vi "Trapezoid Logic.vi"(8 "Total Power":dbl, 9 "Ramp Distance":dbl, 10 "Stop Distance":dbl, 11 "Current \nDistance":dbl(slide) scale=0.0..20.0) -> (2 "Speed":dbl)   [LabVIEW 2013]
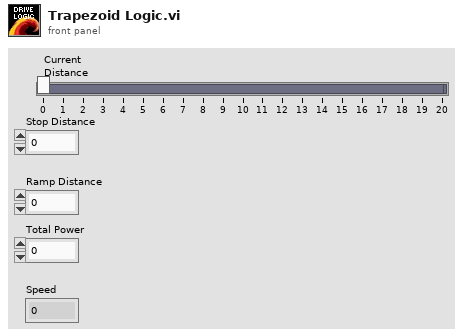
[diagram p1: front panel]
types:
  T1 = enum16{"End Ramp", "Continue Ramp", "Start Ramp"}
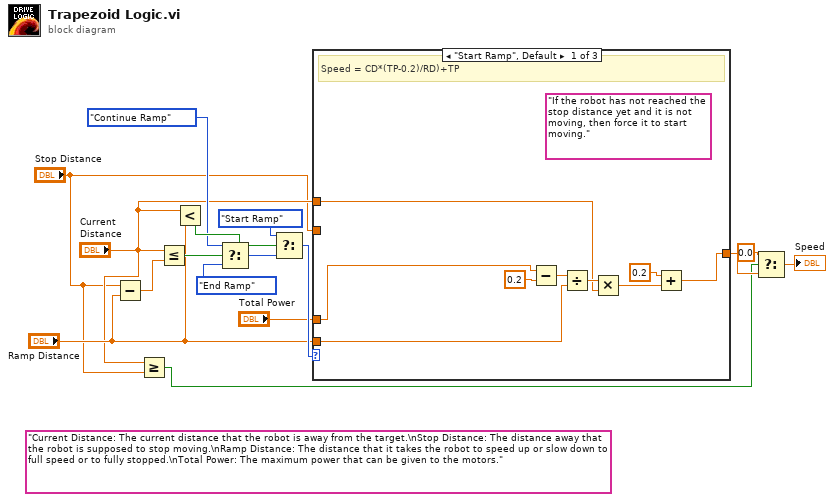
[diagram p0: block diagram]
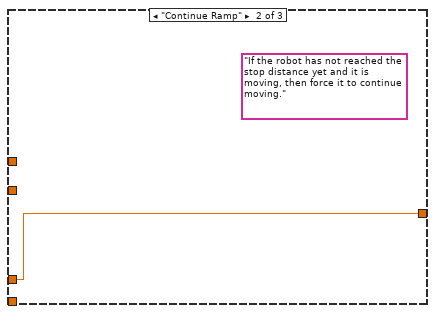
[diagram p2: hidden frame]
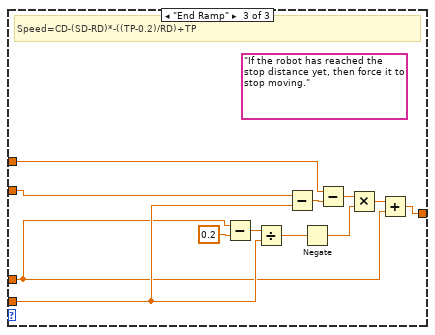
[diagram p3: hidden frame]
diagram:
  (unwired) "Current Distance: The current distance that the robot is away from the target.\nStop Distance: The distance away that the robot is supposed to stop moving.\nRamp Distance: The distance that it takes the robot to speed up or slow down to full speed or to fully stopped.\nTotal Power: The maximum power that can be given to the motors."
  n1 = Subtract(x="Stop Distance", y="Ramp Distance") -> (x-y=w8:dbl)
  n2 = Greater Or Equal?(x="Current \nDistance", y="Stop Distance") -> (x >= y?=w3:bool)
  n3 = Less Or Equal?(x="Current \nDistance", y=w8) -> (x <= y?=w15:bool)
  n4 = Less?(x="Current \nDistance", y="Ramp Distance") -> (x < y?=w16:bool)
  n5 = Select(t=T1."Continue Ramp", s=w15, f=T1."End Ramp") -> (s? t:f=w12:T1)
  n6 = Select(t=T1."Start Ramp", s=w16, f=w12) -> (s? t:f=w13:T1)
  n7 = case shown="\"Start Ramp\", Default" w13 {
    tunnel: "Total Power" -> [w20 w26 w27]
    tunnel: "Current \nDistance" -> [w17 _ w35]
    tunnel: "Ramp Distance" -> [w22 _ w29]
    tunnel: "Stop Distance" -> [_ _ w33]
    tunnel: [w23 w26 w38] -> w4
    frame "Start Ramp", Default {
      (unwired) "If the robot has not reached the stop distance yet and it is not moving, then force it to start moving."
      # "Speed = CD*(TP-0.2)/RD)+TP"
      n8 = Subtract(x=w20, y=0.2) -> (x-y=w18:dbl)
      n9 = Divide(x=w18, y=w22) -> (x/y=w21:dbl)
      n10 = Multiply(x=w21, y=w17) -> (x*y=w25:dbl)
      n11 = Add(x=0.2, y=w25) -> (x+y=w23:dbl)
    }
    frame "Continue Ramp" {
      (unwired) "If the robot has not reached the stop distance yet and it is moving, then force it to continue moving."
    }
    frame "End Ramp" {
      (unwired) "If the robot has reached the stop distance yet, then force it to stop moving."
      # "Speed=CD-(SD-RD)*-((TP-0.2)/RD)+TP"
      n12 = Subtract(x=w27, y=0.2) -> (x-y=w30:dbl)
      n13 = Divide(x=w30, y=w29) -> (x/y=w31:dbl)
      n14 = Subtract(x=w33, y=w29) -> (x-y=w34:dbl)
      n15 = Negate(x=w31) -> (-x=w32:dbl)
      n16 = Subtract(x=w35, y=w34) -> (x-y=w36:dbl)
      n17 = Multiply(x=w36, y=w32) -> (x*y=w37:dbl)
      n18 = Add(x=w37, y=w27) -> (x+y=w38:dbl)
    }
  }
  n19 = Select(t=0.0, s=w3, f=w4) -> (s? t:f=→"Speed":dbl)
